vi "rad_Get Module Programming Modes.vi"(8 "error in (no error)":errorcluster, 11 "Target settings in":T1 {"Primary NIC"."IP Address Request Mode" items=["Static"=1, "DHCP/Link-Local"=2, "Link-Local Only"=4, "DHCP Only"=8]}) -> (0 "error out":errorcluster, 3 "Target settings out":T1 {"Primary NIC"."IP Address Request Mode" items=["Static"=1, "DHCP/Link-Local"=2, "Link-Local Only"=4, "DHCP Only"=8]})   [LabVIEW 2018]
uses:
  Targets/TypeDefs/rad_Target Information.ctl
  Targets/TypeDefs/rad_Target Network Settings.ctl
  <vilib>/nisyscfg/Close (System).vi
  <vilib>/nisyscfg/nisyscfg.lvlib
  <resource>/objmgr/motionsysapi.rc
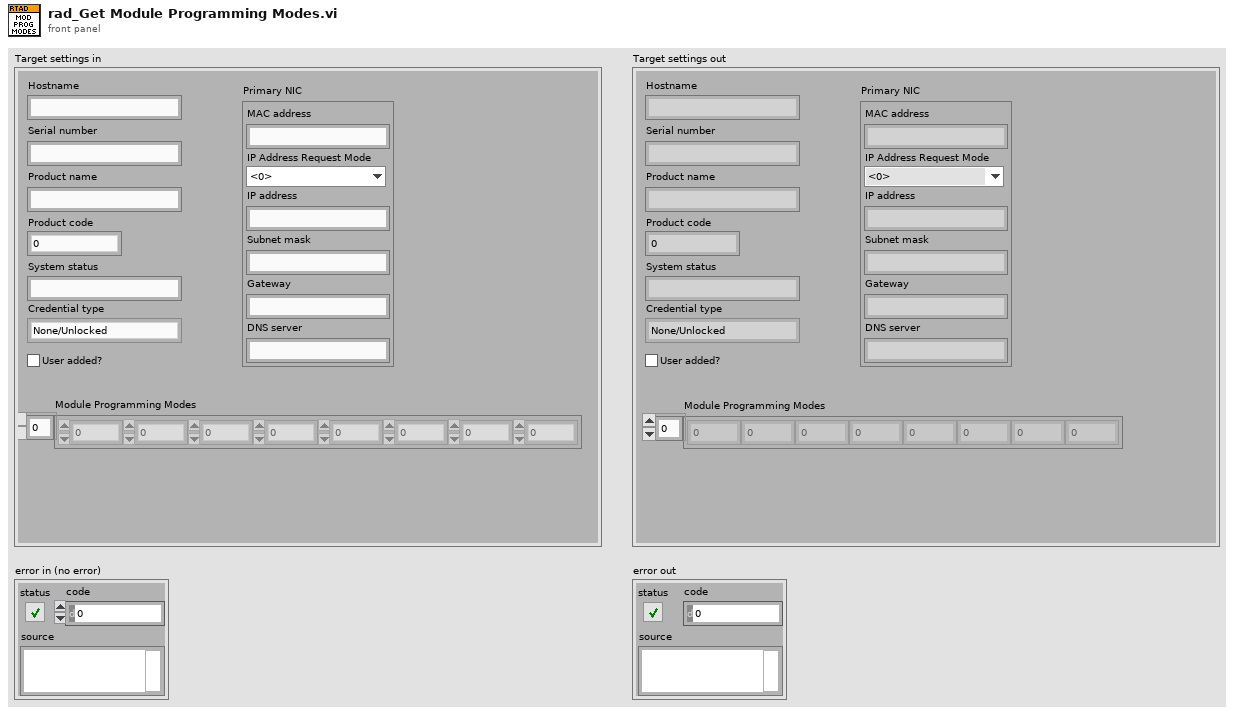
[diagram p1: front panel]
types:
  T1 = typedef "rad_Target Information.ctl" = cluster{"Hostname":string, "Serial number":string, "Product name":string, "Product code":i32, "System status":string, "Credential type":enum16{"None/Unlocked", "FTP Password", "NIAuth Credentials"}, "User added?":bool, "Primary NIC":T2, "Module Programming Modes":dbl[]}
  T2 = typedef "rad_Target Network Settings.ctl" = cluster{"MAC address":string, "IP Address Request Mode":i32, "IP address":string, "Subnet mask":string, "Gateway":string, "DNS server":string}
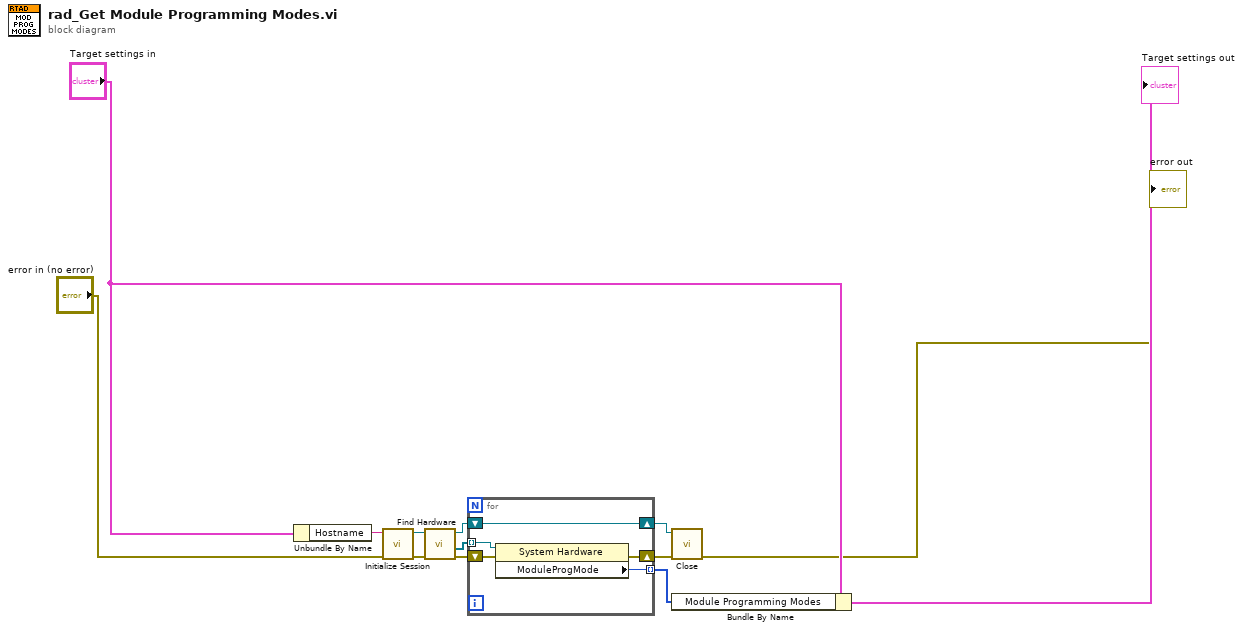
[diagram p0: block diagram]
diagram:
  n1 = Unbundle By Name("Target settings in") -> ("Hostname"=w1:string)
  n2 = call <vilib>:"Initialize Session.vi"("error in (no error)"="error in (no error)", "Target (localhost)"=w1) -> ("error out"=w3:errorcluster, "Session out"=w2:refnum<k21>)  [unwired: 8 in]
  n3 = call <vilib>:"Find Hardware.vi"("error in (no error)"=w3, "Session in"=w2) -> ("error out"=w6:errorcluster, "Resources out"=w5:refnum<k20>[], "Session out"=w4:refnum<k21>)  [unwired: 6 in, 1 out]
  n4 = for {
    tunnel: w5 -> [w18] mode=indexing
    shift-right: [w17] -> w9
    shift-left: w6 -> [w16]
    tunnel: [w15] -> w13 mode=indexing
    shift-right: [w14] -> w8
    shift-left: w4 -> [w14]
    n5 = property class="System Hardware"(reference=w18, error in=w16) -> (error out=w17:errorcluster, "ModuleProgMode"=w15:u32)  [unwired: 1 out]
  }
  n6 = call-poly <vilib>:"Close.vi"("error in (no error)"=w9, "Session in"=w8) -> ("error out"=→"error out":errorcluster)  [unwired: 9 in]
  n7 = Bundle By Name(cluster="Target settings in", "Module Programming Modes"=w13) -> (→"Target settings out":T1)
